vi "Get Robot Tool Position.vi"(8 "error in (no error)":errorcluster, 11 "UR5 Robot in":refnum<class "UR5 Robot.lvclass">) -> (0 "error out":errorcluster, 2 "Tool Pose":string, 3 "UR5 Robot out":refnum<class "UR5 Robot.lvclass">)   [LabVIEW 2018, in "UR5 Robot.lvlib" / "UR5 Robot.lvclass"]
uses:
  UR5 Robot.lvclass
  UR5 Robot.lvclass/UR5 Robot.ctl
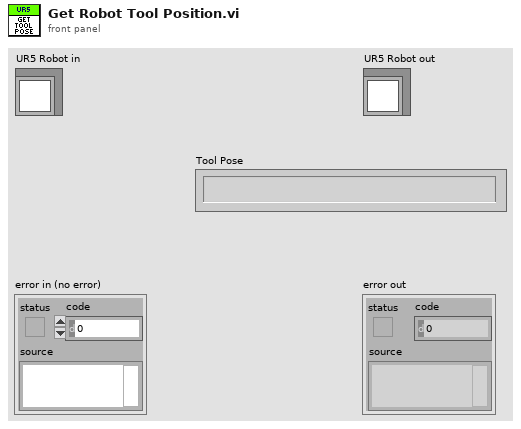
[diagram p1: front panel]
types:
  T1 = enum16{"Standard", "Buffered", "CRLF", "Immediate"}
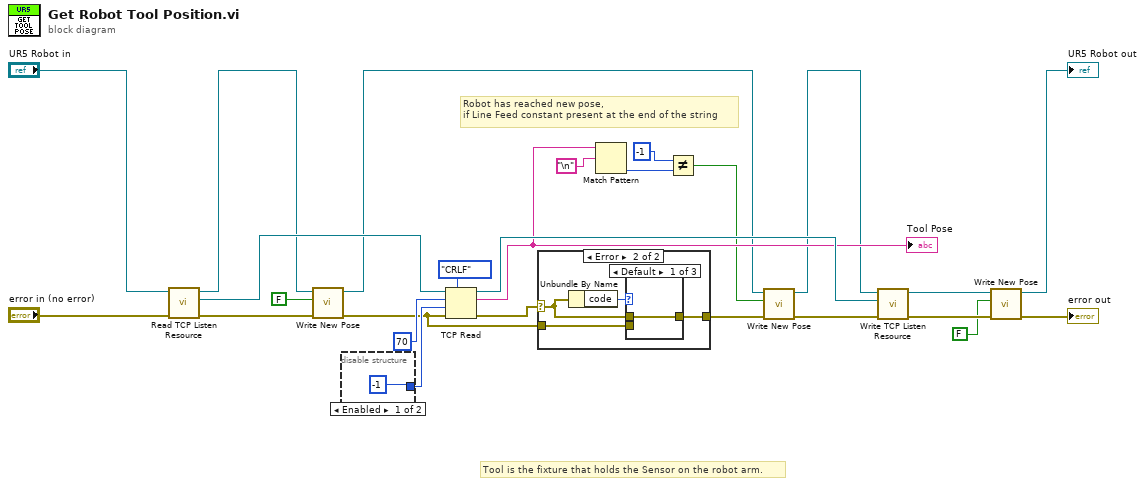
[diagram p0: block diagram]
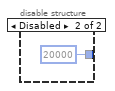
[diagram p2: hidden frame]
diagram:
  # "Robot has reached new pose,\nif Line Feed constant present at the end of the string"
  # "Tool is the fixture that holds the Sensor on the robot arm."
  n1 = call "Read TCP Listen Resource.vi"("error in (no error)"="error in (no error)", "UR5 Robot in"="UR5 Robot in") -> ("error out"=w24:errorcluster, "TCP Listen Resource"=w23:refnum<k5>, "UR5 Robot out"=w17:refnum<class "UR5 Robot.lvclass">)  [unwired: 7 in]
  n2 = call "Write New Pose.vi"("error in (no error)"=w24, "New Pose?"=FALSE, "UR5 Robot in"=w17) -> ("error out"=w3:errorcluster, "UR5 Robot out"=w2:refnum<class "UR5 Robot.lvclass">)  [unwired: 7 in]
  n3 = disable-structure shown="Enabled" {
    disable-tunnel: [-1 ("timeout ms (25000)") 20000 ("timeout ms (25000)")] -> w10
    frame Enabled {
    }
    frame Disabled {
    }
  }
  n4 = TCP Read(connection ID=w23, bytes to read=70, error in (no error)=w3, 7:T1."CRLF" ("mode (standard)"), 9:w10) -> (connection ID out=w21:refnum<k5>, data out=w18:string, error out=w9:errorcluster)
  "Tool Pose" <- w18
  n5 = case shown="Error" w9 {
    selector: w9 -> [w29 w32]
    tunnel: [w29 w30] -> w8
    tunnel: w3 -> [_ w31]
    frame No Error {
    }
    frame Error {
      n6 = Unbundle By Name(w32) -> ("code"=w33:i32)
      n7 = case shown="Default" w33 {
        tunnel: w32 -> [w34 _ _]
        tunnel: w31 -> [_ w35 w36]
        tunnel: [w34 w35 w36] -> w30
        frame Default {
        }
        frame 56 {
        }
        frame 66 {
        }
      }
    }
  }
  n8 = Match Pattern(string=w18, regular expression="\n") -> (offset past match=w6:i32)  [unwired: 1 in, 3 out]
  n9 = Not Equal?(x=-1, y=w6) -> (x != y?=w4:bool)
  n10 = call "Write New Pose.vi"("error in (no error)"=w8, "New Pose?"=w4, "UR5 Robot in"=w2) -> ("error out"=w22:errorcluster, "UR5 Robot out"=w16:refnum<class "UR5 Robot.lvclass">)  [unwired: 7 in]
  n11 = call "Write TCP Listen Resource.vi"("error in (no error)"=w22, "TCP Listen Resource"=w21, "UR5 Robot in"=w16) -> ("error out"=w20:errorcluster, "UR5 Robot out"=w19:refnum<class "UR5 Robot.lvclass">)  [unwired: 7 in]
  n12 = call "Write New Pose.vi"("error in (no error)"=w20, "New Pose?"=FALSE, "UR5 Robot in"=w19) -> ("error out"=→"error out":errorcluster, "UR5 Robot out"=→"UR5 Robot out":refnum<class "UR5 Robot.lvclass">)  [unwired: 7 in]
